vi "simx Call Script Function.vi"(0 "clientID":i32, 1 "scriptDescription":string, 2 "options":i32, 3 "functionName":string, 4 "inIntCnt":i32, 5 "inInt":i32, 6 "inFloatCnt":i32, 7 "error in (no error)":errorcluster, 8 "inFloat":sgl, 9 "inStringCnt":i32, 10 "inString":string, 11 "inBufferSize":i32, 12 "inBuffer":string, 13 "outIntCnt":i32, 14 "outInt":i32, 15 "outFloatCnt":i32, 16 "outFloat":sgl, 17 "outStringCnt":i32, 18 "outString":string, 19 "outBufferSize":i32, 25 "operationMode":i32, 26 "outBuffer":string) -> (20 "outIntCnt out":i32, 21 "outInt out":i32, 22 "outFloatCnt out":i32, 23 "outFloat out":sgl, 24 "outStringCnt out":i32, 27 "error out":errorcluster)   [LabVIEW 2019, in "PXL_V-REP.lvlib"]
doc: "EXTAPI_DLLEXPORT simxInt simxCallScriptFunction(simxInt clientID,const simxChar* scriptDescription,simxInt options,const simxChar* functionName,simxInt inIntCnt,const simxInt* inInt,simxInt inFloatCnt,const simxFloat* inFloat,simxInt inStringCnt,const simxChar* inString,simxInt inBufferSize,const simxUChar* inBuffer,simxInt* outIntCnt,simxInt** outInt,simxInt* outFloatCnt,simxFloat** outFloat,simxInt* outStringCnt,simxChar** outString,simxInt* outBufferSize,simxUChar** outBuffer,simxInt operationMode);"
uses:
  PXL_V-REP.lvlib
  <userlib>/V-REP/remoteApi.dll
panel:
  out "outBuffer out":string
  out "outBufferSize out":i32
  out "outString out":string
  out "function return":i32
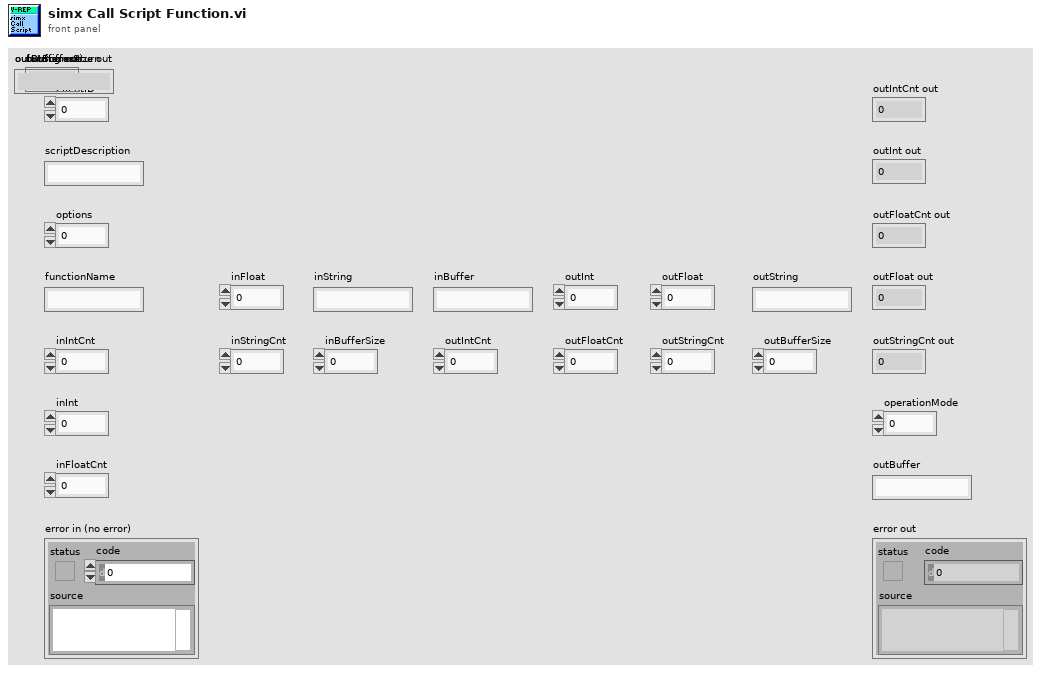
[diagram p1: front panel]
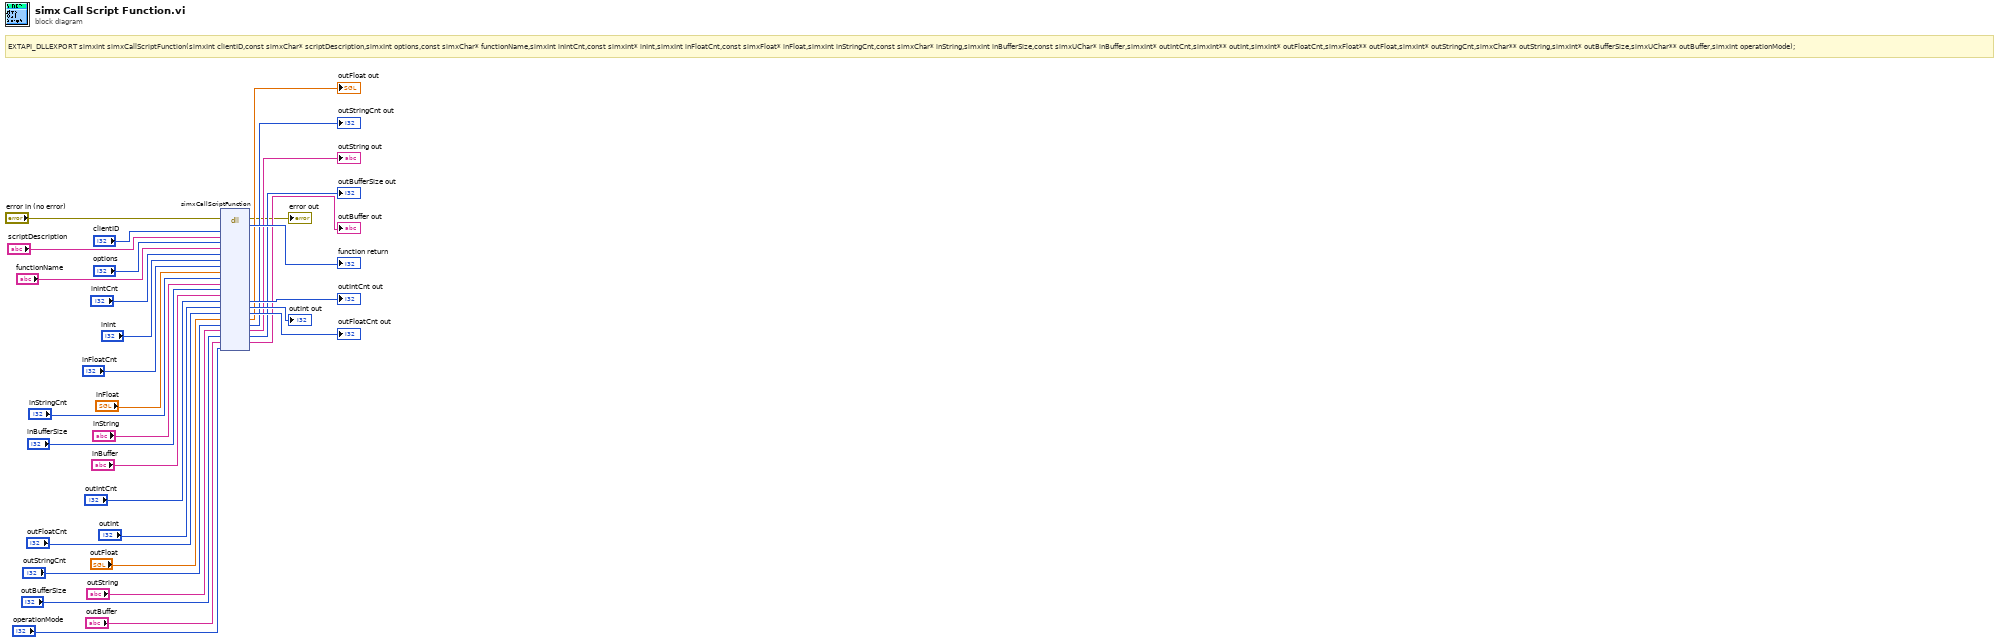
[diagram p0: block diagram]
diagram:
  # "EXTAPI_DLLEXPORT simxInt simxCallScriptFunction(simxInt clientID,const simxChar* scriptDescription,simxInt options,const simxChar* functionName,simxInt inIntCnt,const simxInt* inInt,simxInt inFloatCnt,const simxFloat* inFloat,simxInt inStringCnt,const simxChar* inString,simxInt inBufferSize,const simxUChar* inBuffer,simxInt* outIntCnt,simxInt** outInt,simxInt* outFloatCnt,simxFloat** outFloat,simxInt* outStringCnt,simxChar** outString,simxInt* outBufferSize,simxUChar** outBuffer,simxInt operationMode);"
  n1 = dll-call lib="C:/Program Files (x86)/National Instruments/LabVIEW 2019/user.lib/V-REP/remoteApi.*" fn="simxCallScriptFunction"(error in="error in (no error)", "clientID"="clientID", "scriptDescription"="scriptDescription", "options"="options", "functionName"="functionName", "inIntCnt"="inIntCnt", "inInt"="inInt", "inFloatCnt"="inFloatCnt", "inFloat"="inFloat", "inStringCnt"="inStringCnt", "inString"="inString", "inBufferSize"="inBufferSize", "inBuffer"="inBuffer", "outIntCnt"="outIntCnt", "outInt"="outInt", "outFloatCnt"="outFloatCnt", "outFloat"="outFloat", "outStringCnt"="outStringCnt", "outString"="outString", "outBufferSize"="outBufferSize", "outBuffer"="outBuffer", "operationMode"="operationMode") -> (error out=→"error out":errorcluster, →"function return":i32, "outIntCnt"=→"outIntCnt out":i32, "outInt"=→"outInt out":i32, "outFloatCnt"=→"outFloatCnt out":i32, "outFloat"=→"outFloat out":sgl, "outStringCnt"=→"outStringCnt out":i32, "outString"=→"outString out":string, "outBufferSize"=→"outBufferSize out":i32, "outBuffer"=→"outBuffer out":string)  [unwired: 15 in, 1 out]
